vi "S2C_CMD_FindCmd.vi"(8 "Error In":errorcluster, 11 "Index":i32) -> (0 "Error Out":errorcluster, 1 "Returns":string[](array[string]), 2 "Parameters":string[][](array[string]), 3 "AllCmds":string[](array[string]))   [LabVIEW 2015]
doc: "Find the parameters associated with a command, given the command index."
uses:
  S2C_CMD_Globals.vi
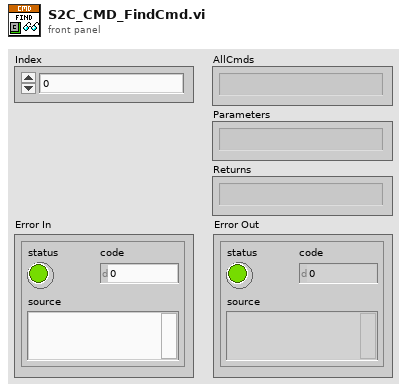
[diagram p1: front panel]
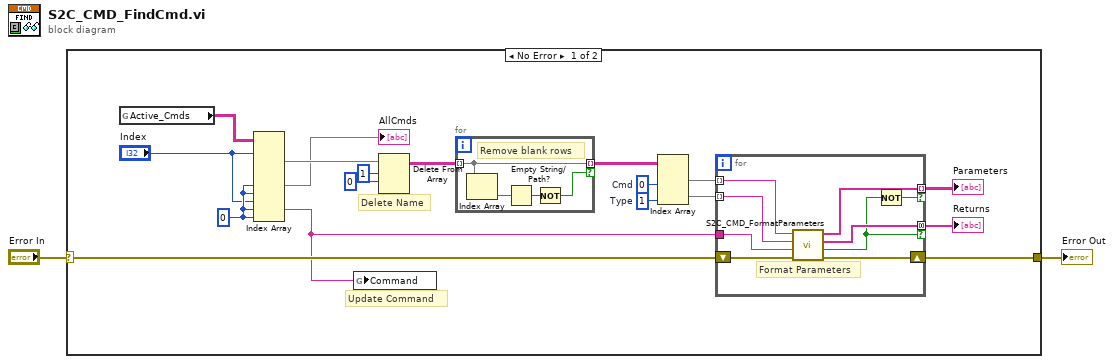
[diagram p0: block diagram]
diagram:
  n1 = case shown="No Error" "Error In" {
    selector: "Error In" -> [w14 w34]
    tunnel: [w13 w34] -> w1
    frame No Error {
      w9 = 0 ("index (col)")
      w11 = 1  # Type
      w17 = 0  # Cmd
      # "Update Command"
      # "Delete Name"
      n2 = global read "S2C_CMD_Globals.vi" "Active_Cmds"() -> (w6:string[][][])
      n3 = Index Array(array=w6, index (dim 0) #1="Index", index (dim 1) #2=w9, index (dim 2) #2=w9, index (dim 0) #3="Index", index (dim 1) #3=w9, index (dim 2) #3=w9) -> (element #1=w20:string[][], element #2=→"AllCmds":string[], element #3=w4:string)  [unwired: 3 in]
      n4 = global write "S2C_CMD_Globals.vi" "Command"(w4) -> ()
      n5 = Delete From Array(array=w20, length=1, index (row)=0) -> (array with subset deleted=w8:string[][])  [unwired: 1 in, 1 out]
      n6 = for {
        tunnel: w8 -> [w24] mode=indexing
        tunnel: [w24] -> w7 mode=indexing if=w21
        # "Remove blank rows"
        n7 = Index Array(array=w24) -> (element=w23:string)  [unwired: 1 in]
        n8 = Empty String/Path?(string/path=w23) -> (empty?=w22:bool)
        n9 = Not(x=w22) -> (.not. x?=w21:bool)
      }
      n10 = Index Array(array=w7, index (col) #1=w17, index (col) #2=w11) -> (element #1=w16:string[], element #2=w15:string[])  [unwired: 2 in]
      n11 = for {
        shift-right: [w28] -> w13
        shift-left: w14 -> [w32]
        tunnel: w16 -> [w29] mode=indexing
        tunnel: w15 -> [w30] mode=indexing
        tunnel: w4 -> [w31]
        tunnel: [w26] -> w12 mode=indexing if=w33
        tunnel: [w27] -> w5 mode=concatenating if=w25
        # "Format Parameters"
        n12 = call "S2C_CMD_FormatParameters.vi"("Error In"=w32, "CmdName"=w31, "Type"=w30, "Cmd"=w29) -> ("Error Out"=w28:errorcluster, "RecReturn?"=w25:bool, "Returns"=w27:string[], "Parameters"=w26:string[])  [unwired: 4 in]
        n13 = Not(x=w25) -> (.not. x?=w33:bool)
      }
      "Parameters" <- w12
      "Returns" <- w5
    }
    frame Error {
    }
  }
  "Error Out" <- w1
